vi "myRIO_BRig_RT_comm_webdav_endExp_storeData.vi"(9 "input_fileName_prefix":string, 11 "input_hSession":T1) -> (3 "output_hSession":T1)   [LabVIEW 2014]
uses:
  <vilib>/WebDAVClient/NI_WebDAV.lvlib
  <vilib>/WebDAVClient/Advanced/SessionHandle.ctl
panel:
  out "date string":string
  out "code":i32
  out "error out":errorcluster
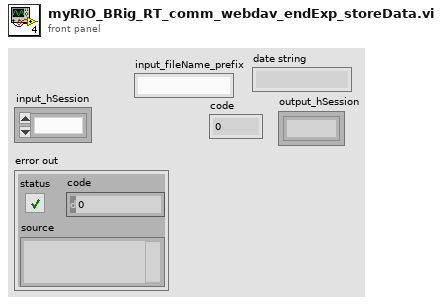
[diagram p1: front panel]
types:
  T1 = typedef "NI_WebDAV.lvlib/SessionHandle.ctl" = refnum<k1>
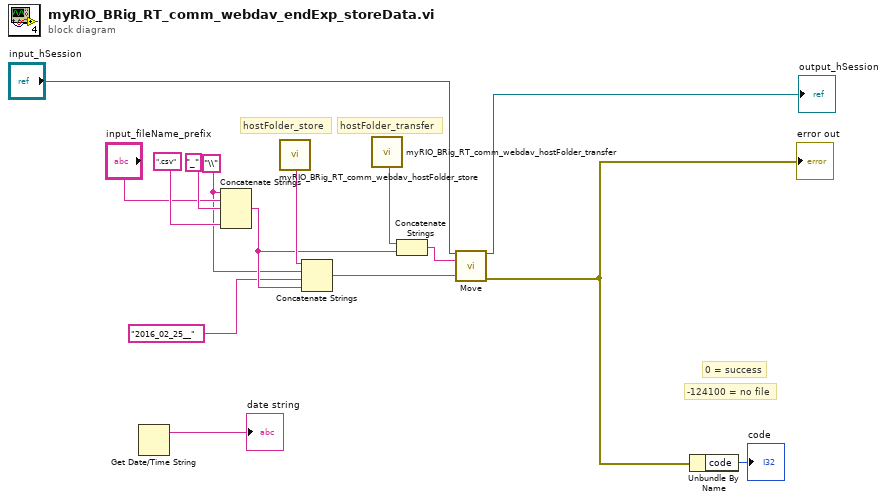
[diagram p0: block diagram]
diagram:
  w6 = "\\" ("string")
  # "-124100 = no file"
  # "0 = success"
  # "hostFolder_store"
  # "hostFolder_transfer"
  n1 = Get Date/Time String() -> (date string=→"date string":string)  [unwired: 3 in, 1 out]
  n2 = Concatenate Strings(w6, "input_fileName_prefix", "_" ("string"), ".csv" ("string")) -> (w7:string)  [unwired: 1 in]
  n3 = call "myRIO_BRig_RT_comm_webdav_hostFolder_store.vi"() -> ("output_HostFolder"=w12:string)  [unwired: 11 in]
  n4 = Concatenate Strings(w12, w6, "2016_02_25__" ("string"), w7) -> (w10:string)
  n5 = call "myRIO_BRig_RT_comm_webdav_hostFolder_transfer.vi"() -> ("output_HostFolder"=w13:string)  [unwired: 11 in]
  n6 = Concatenate Strings(w13, w7) -> (w11:string)
  n7 = call <vilib>:"Move.vi"("session handle"="input_hSession", "relative source uri"=w11, "relative destination uri"=w10) -> ("session handle out"=→"output_hSession":T1, "error out"=w4:errorcluster)  [unwired: 11 in]
  "error out" <- w4
  n8 = Unbundle By Name(w4) -> ("code"=→"code":i32)
